vi "ActionVIOnCompile.vi"(8 "error in (no error)":errorcluster, 11 "Device Item Ref in":T1 format="%.0x") -> (0 "error out":errorcluster)   [LabVIEW 2021, in "DAQ Analog InOut System Explorer.lvlib"]
uses:
  DAQ Analog InOut System Explorer.lvlib
  <vilib>/NI VeriStand/Custom Device API/Custom Device Item Ref.ctl
  Shared/Compiled.Settings.ctl
  Types/Output Channel Parameters.ctl
  Types/Input Channel Parameters.ctl
  Shared/Constants.vi
  <vilib>/NI VeriStand/Custom Device API/Get Item Property (Double).vi
  <vilib>/NI VeriStand/Custom Device API/Set Item Property (Variant).vi
  <vilib>/NI VeriStand/Custom Device API/Custom Device API.lvlib
  <vilib>/NI/NIVS Inline Async API/_Data Access System Explorer/Data Access System Explorer.lvlib
  Shared/DAQ Analog InOut Shared.lvlib
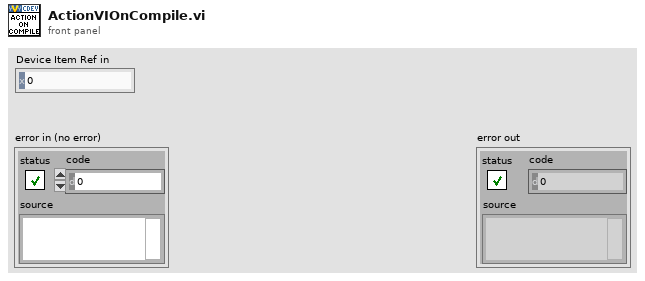
[diagram p1: front panel]
types:
  T1 = typedef "Custom Device API.lvlib/Custom Device Item Ref.ctl" = u64
  T2 = typedef "DAQ Analog InOut Shared.lvlib/Compiled.Settings.ctl" = cluster{"Name":string, "AO Enable":bool, "AI Enable":bool, "Main Page Parameters":cluster{"AI Channels Used":u8, "AO Channels Used":u8, "Select channel type to add":string, "Device Name in Max":string, "PCL Decimation":u16, "Async Timeout (ms)":u16}, "Output Channel Parameters":T3, "AI Signals properties Array":T4[], "AI Sample Rate":dbl, "PCL Rate [Hz]":dbl}
  T3 = typedef "DAQ Analog InOut System Explorer.lvlib/Output Channel Parameters.ctl" = cluster{"AO MaxV":dbl, "AO MinV":dbl}
  T4 = typedef "DAQ Analog InOut System Explorer.lvlib/Input Channel Parameters.ctl" = cluster{"AI MaxV":dbl, "AI MinV":dbl, "Input Configuration":u16}
  T5 = typedef "Custom Device API.lvlib/Custom Device Item Info.ctl" = cluster{"Name":string, "Is Channel":bool, "GUID":string, "Is Waveform":bool}
  T6 = typedef "DAQ Analog InOut System Explorer.lvlib/Main Page Parameters.ctl" = cluster{"AI Channels Used":u8, "AO Channels Used":u8, "Select channel type to add":string, "Device Name in Max":string, "PCL Decimation":u16, "Async Timeout (ms)":u16}
  T7 = cluster{"Name":string, "Type":enum16{"Output/Write", "Input/Read", "Input/ReadWrite"}, "VS Refs":T1[]}[]
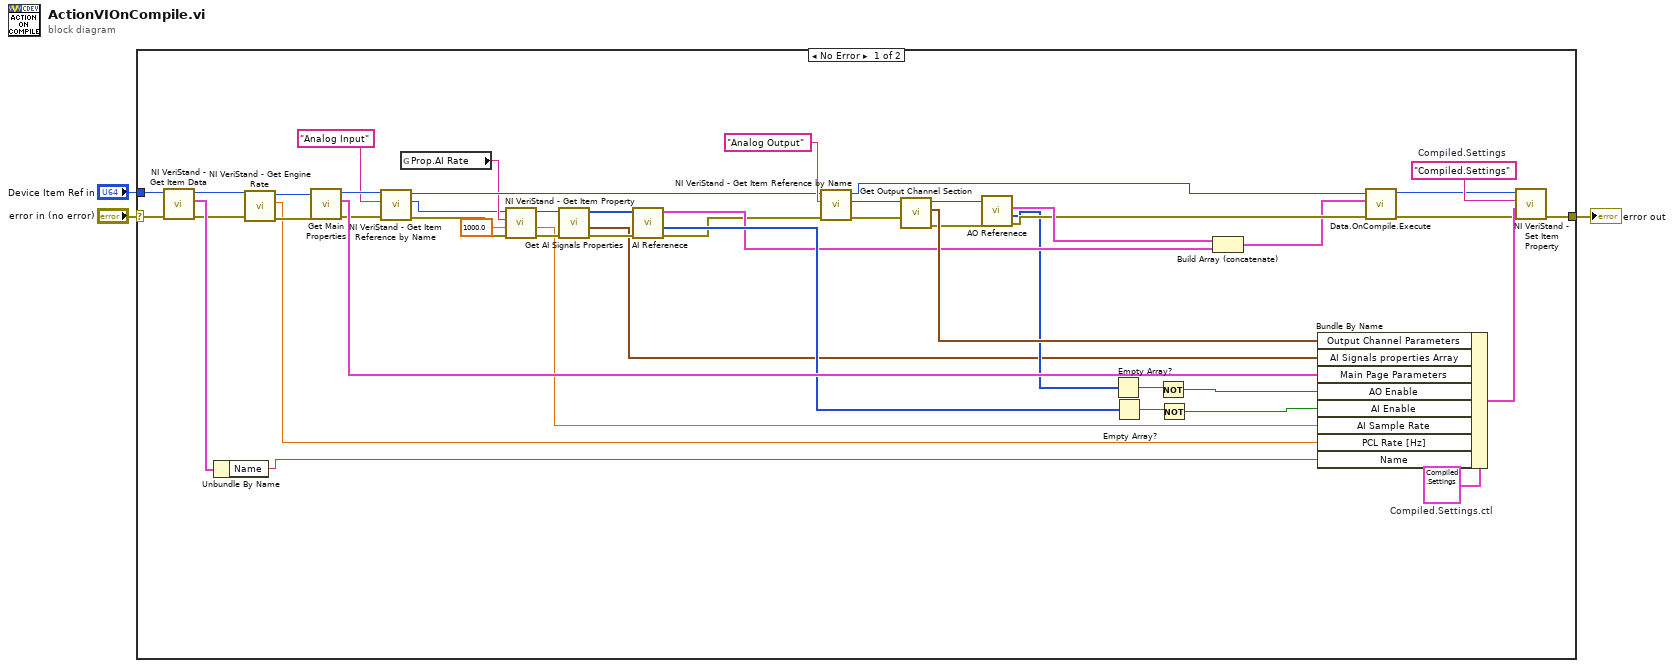
[diagram p0: block diagram]
diagram:
  n1 = case shown="No Error" "error in (no error)" {
    selector: "error in (no error)" -> [w48 w52]
    tunnel: [w49 w52] -> w2
    tunnel: "Device Item Ref in" -> [w47 _]
    frame No Error {
      w43 = T2 {"Name"="", "AO Enable"=FALSE, "AI Enable"=FALSE, "Main Page Parameters"={"AI Channels Used"=0, "AO Channels Used"=0, "Select channel type to add"="", "Device Name in Max"="PXI1Slot2", "PCL Decimation"=0, "Async Timeout (ms)"=0}, "Output Channel Parameters"={"AO MaxV"=0.0, "AO MinV"=0.0}, "AI Signals properties Array"=[], "AI Sample Rate"=0.0, "PCL Rate [Hz]"=0.0}  # Compiled.Settings.ctl
      w51 = "Compiled.Settings"  # Compiled.Settings
      n2 = call <vilib>:"NI VeriStand - Get Item Data.vi"("error in (no error)"=w48, "Item Ref in"=w47) -> ("error out"=w7:errorcluster, "Item Info"=w46:T5, "Item Ref out"=w8:T1)  [unwired: 6 in, 1 out]
      n3 = Unbundle By Name(w46) -> ("Name"=w9:string)
      n4 = call <vilib>:"NI VeriStand - Get Engine Rate.vi"("error in (no error)"=w7, "Item Ref in"=w8) -> ("error out"=w6:errorcluster, "Rate (Hz)"=w4:dbl, "Item Ref out"=w5:T1)  [unwired: 7 in]
      n5 = call "Get Main Properties.vi"("error in (no error)"=w6, "Ref in"=w5) -> ("error out"=w36:errorcluster, "Main Page Parameters"=w38:T6, "Ref out"=w37:T1)  [unwired: 7 in]
      n6 = call <vilib>:"NI VeriStand - Get Item Reference by Name.vi"("error in (no error)"=w36, "Item Name"="Analog Input", "Parent Ref in"=w37) -> ("error out"=w15:errorcluster, "Item Ref"=w13:T1, "Parent Ref out"=w29:T1)  [unwired: 5 in, 1 out]
      n7 = global read "Constants.vi" "Prop.AI Rate"() -> (w16:string)
      n8 = call-poly <vilib>:"NI VeriStand - Get Item Property.vi"("error in (no error)"=w15, "Default Value"=1000.0, "Property Name"=w16, "Item Ref in"=w13) -> ("error out"=w14:errorcluster, "Value"=w11:dbl, "Item Ref out"=w12:T1)  [unwired: 4 in, 1 out]
      n9 = call "Get AI Signals Properties.vi"("error in (no error)"=w14, "Item Ref in"=w12) -> ("error out"=w19:errorcluster, "AI Signal properties Array"=w17:T4[], "AI Signal Refs"=w20:T1[])  [unwired: 7 in]
      n10 = call "AI Referenece.vi"("error in (no error)"=w19, "Child Refs"=w20) -> ("error in (no error) 2"=w18:errorcluster, 1:"AI Refs"=w30:T1[], 3:"AI Refs"=w26:T7)  [unwired: 7 in]
      n11 = call <vilib>:"NI VeriStand - Get Item Reference by Name.vi"("error in (no error)"=w18, "Item Name"="Analog Output", "Parent Ref in"=w29) -> ("error out"=w33:errorcluster, "Item Ref"=w32:T1, "Parent Ref out"=w24:T1)  [unwired: 5 in, 1 out]
      n12 = call "Get Output Channel Section.vi"("error in (no error)"=w33, "Ref in"=w32) -> ("error out"=w27:errorcluster, "Output Channel Parameters"=w31:T3, "Ref out"=w28:T1)  [unwired: 7 in]
      n13 = call "AO Referenece.vi"("error in (no error)"=w27, "Item Ref in"=w28) -> ("error out"=w23:errorcluster, 1:"AO Refs"=w22:T1[], 2:"AO Refs"=w25:T7)  [unwired: 6 in, 1 out]
      n14 = Empty Array?(array=w22) -> (empty?=w42:bool)
      n15 = Empty Array?(array=w30) -> (empty?=w41:bool)
      n16 = Not(x=w42) -> (.not. x?=w39:bool)
      n17 = Not(x=w41) -> (.not. x?=w40:bool)
      n18 = Build Array (concatenate)(w25, w26) -> (w21:T7)
      n19 = Bundle By Name(cluster=w43, "Output Channel Parameters"=w31, "AI Signals properties Array"=w17, "Main Page Parameters"=w38, "AO Enable"=w39, "AI Enable"=w40, "AI Sample Rate"=w11, "PCL Rate [Hz]"=w4, "Name"=w9) -> (w50:T2)
      n20 = call <vilib>:"Data.OnCompile.Execute.vi"("error in"=w23, "VS Ref Groups"=w21, "Custom Device Ref"=w24) -> ("error out"=w45:errorcluster, "Custom Device Ref"=w44:T1)  [unwired: 7 in]
      n21 = call-poly <vilib>:"NI VeriStand - Set Item Property.vi"("error in (no error)"=w45, "Value"=w50, "Property Name"=w51, "Item Ref in"=w44) -> ("error out"=w49:errorcluster)  [unwired: 5 in, 2 out]
    }
    frame Error {
    }
  }
  "error out" <- w2
